vi "Read Configuration Class Name.vi"(8 "error in":errorcluster, 11 "Scan Engine editor node in":refnum<class "Scan Engine editor node.lvclass">) -> (0 "error out":errorcluster, 2 "Class Name":string, 3 "Scan Engine editor node out":refnum<class "Scan Engine editor node.lvclass">)   [LabVIEW 2013, in "Scan Engine editor node.lvclass"]
uses:
  Scan Engine editor node.lvclass
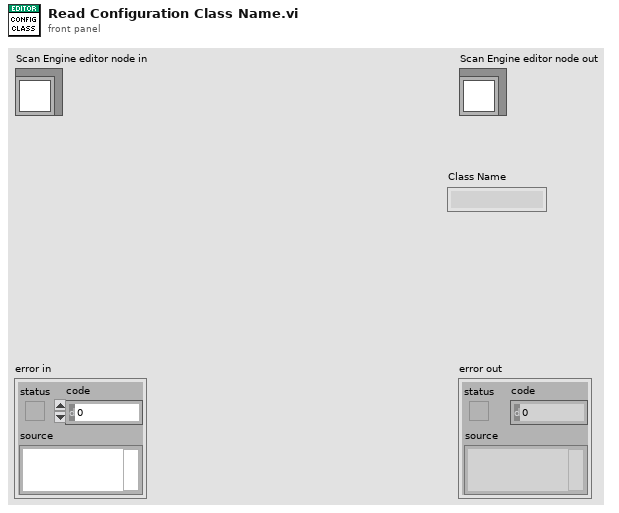
[diagram p1: front panel]
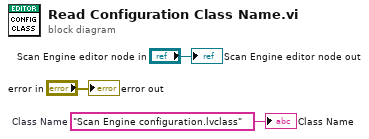
[diagram p0: block diagram]
diagram:
  w1 = "Scan Engine configuration.lvclass"  # Class Name
  "error out" <- "error in"
  "Scan Engine editor node out" <- "Scan Engine editor node in"
  "Class Name" <- w1
